vi "创建数组.vi"() -> ()   [LabVIEW 2018]
panel:
  in  "停止":bool
  out "字符串":string
  in  "数组":dbl[][][](array[numeric])
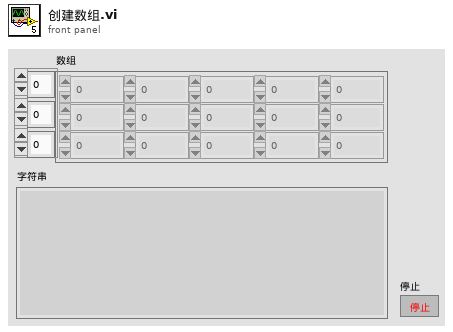
[diagram p1: front panel]
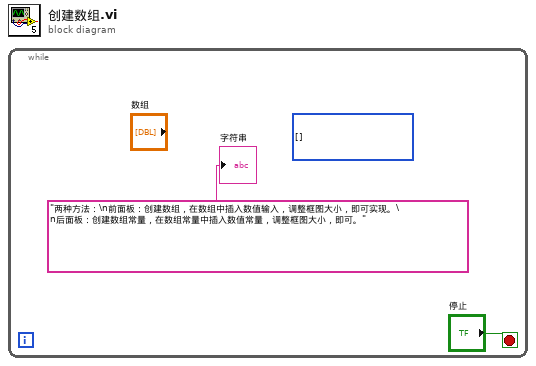
[diagram p0: block diagram]
diagram:
  n1 = while {
    stop <- "停止" stop-if-true
    (unwired) i32[][] []
    "字符串" <- "两种方法：\n前面板：创建数组，在数组中插入数值输入，调整框图大小，即可实现。\n后面板：创建数组常量，在数组常量中插入数值常量，调整框图大小，即可。"
  }
